vi "GetDocument.vi"(0 "reference in":refnum<class "DP_WebView.lvclass">, 5 "Error In":errorcluster) -> (14 "reference out":refnum<class "DP_WebView.lvclass">, 15 "Result":string, 19 "Error Out":errorcluster)   [LabVIEW 2020, in "DP_WebView.lvclass"]
doc: "Get HTML comtent"
uses:
  DP_WebView.lvclass
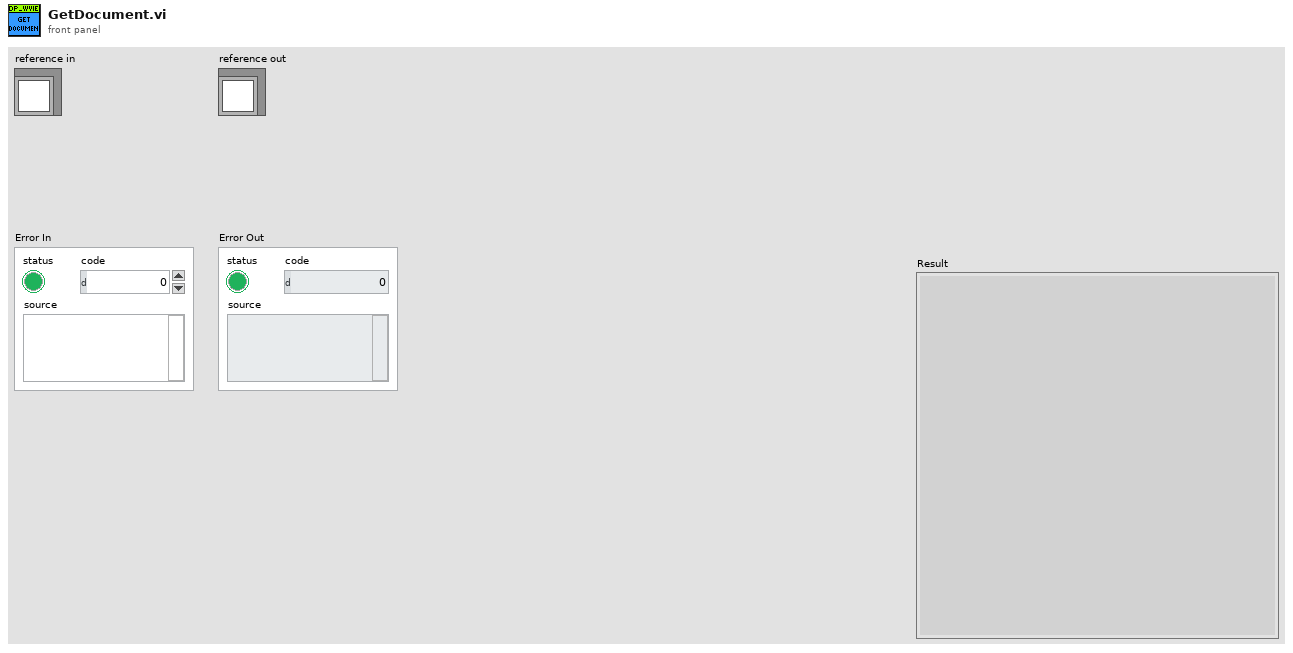
[diagram p1: front panel]
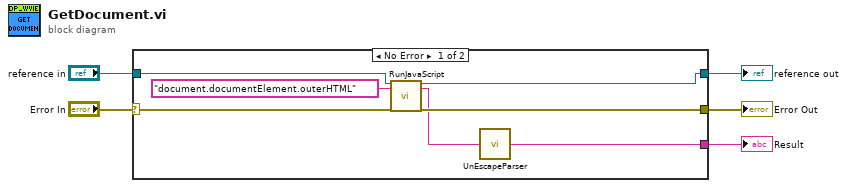
[diagram p0: block diagram]
diagram:
  n1 = case shown="No Error" "Error In" {
    selector: "Error In" -> [w10 w14]
    tunnel: [w8 w14] -> w4
    tunnel: [w9 w13] -> w2
    tunnel: "reference in" -> [w12 w13]
    tunnel: [w6 _] -> w1
    frame No Error {
      n2 = call-dynamic "RunJavaScript.vi"("reference in"=w12, "Java Script Function"="document.documentElement.outerHTML" ("javaScript"), "Error In"=w10) -> ("reference out"=w9:refnum<class "DP_WebView.lvclass">, "Result"=w7:string, "Error Out"=w8:errorcluster)  [unwired: 13 in, 1 out]
      n3 = call "UnEscapeParser.vi"("String In"=w7) -> ("String Out"=w6:string)
    }
    frame Error {
    }
  }
  "Error Out" <- w4
  "reference out" <- w2
  "Result" <- w1
